vi "Global Variables.vi"() -> ()   [LabVIEW 2020]
panel:
  in  "vision Yangle":dbl
  in  "shooter velocity":dbl
  in  "vision distance":dbl
  in  "vision Xangle":dbl
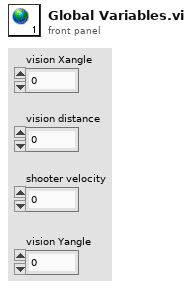
[diagram p1: front panel]
diagram:
